vi "Throw.vi"(0 "exception":refnum<class "Exception.lvclass">, 11 "output cluster":errorcluster) -> (4 "exception out":refnum<class "Exception.lvclass">, 15 "error out":errorcluster)   [LabVIEW 2015, in "LV Exceptions v1.lvlib" / "Exception.lvclass"]
doc: "Inserts exception object into error cluster."
uses:
  Exception.lvclass
  Exception Error Code.ctl
  LV Exceptions v1.lvlib
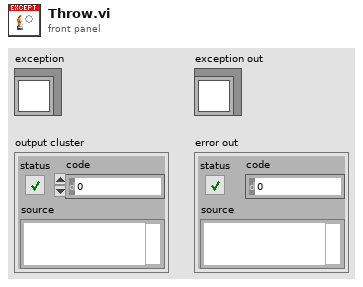
[diagram p1: front panel]
types:
  T1 = typedef "LV Exceptions v1.lvlib/Exception.lvclass/Exception Error Code.ctl" = i32
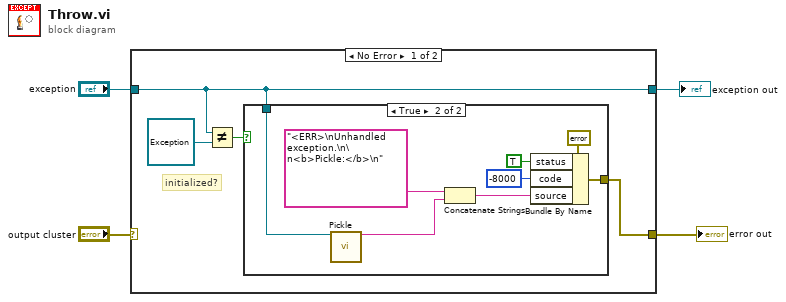
[diagram p0: block diagram]
diagram:
  n1 = case shown="No Error" "output cluster" {
    selector: "output cluster" -> [_ w18]
    tunnel: [w8 w18] -> w4
    tunnel: [w6 w17] -> w2
    tunnel: "exception" -> [w6 w17]
    frame No Error {
      # "initialized?"
      n2 = Not Equal?(x=w6, y=refnum<class "Exception.lvclass"> refnum ("exception")) -> (x != y?=w5:bool)
      n3 = case shown="True" w5 {
        tunnel: [_ w13] -> w8
        tunnel: w6 -> [_ w9]
        frame False {
        }
        frame True {
          n4 = call "Pickle.vi"("variant"=w9) -> ("pickle"=w10:string)  [unwired: 14 in]
          n5 = Concatenate Strings("<ERR>\nUnhandled exception.\n\n<b>Pickle:</b>\n" ("format string"), w10) -> (w15:string)
          n6 = Bundle By Name(cluster=errorcluster {"status"=FALSE, "code"=0, "source"=""} ("error IO"), "status"=TRUE, "code"=T1 -8000 ("y"), "source"=w15) -> (w13:errorcluster)
        }
      }
    }
    frame Error {
    }
  }
  "error out" <- w4
  "exception out" <- w2
